vi "Stop.vi"(8 "error in (no error)":errorcluster, 11 "Topic Actor Stop Command in":refnum<class "Topic Actor Stop Command.lvclass">) -> (0 "error out":errorcluster, 2 "Stop?":bool, 3 "Topic Actor Stop Command out":refnum<class "Topic Actor Stop Command.lvclass">)   [LabVIEW 2016, in "Stream Mediator.lvlib" / "Topic Actor Stop Command.lvclass"]
doc: "--\nCopyright © 2017 Composed SystemsI All rights reserved.\n\nAuthor: Jon McBee <jon.mcbee@composed.io>\n\nThis library is provided \"AS IS\" ,WITHOUT WARRANTIES OR\nCONDITIONS OF ANY KIND, either express or implied.\n\nComposed Systems -- composed.io\n\nStream 0.0.1.1\nJon McBee - Composed Systems\nCopyright (c) 2017, Composed Systems"
uses:
  <userlib>/Composed Systems/Stream/Mediator/Classes/Topic Actor Stop Command/Topic Actor Stop Command.lvclass
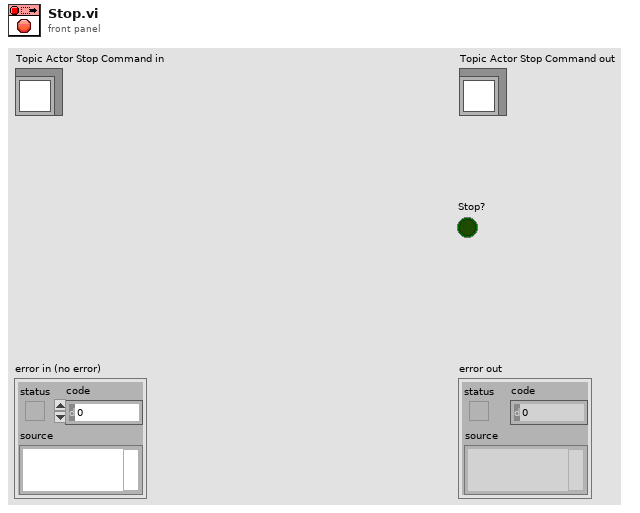
[diagram p1: front panel]
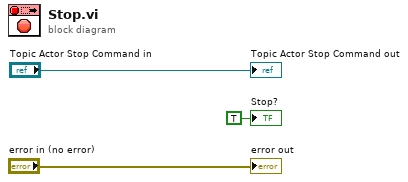
[diagram p0: block diagram]
diagram:
  "error out" <- "error in (no error)"
  "Topic Actor Stop Command out" <- "Topic Actor Stop Command in"
  "Stop?" <- TRUE ("Stop?")
